vi "ConvertTEDtoWFM.vi"(9 "TED Status":T2[](array[typedef])=[{"Output"=FALSE, "SetPoint"=0.0, "Temperature"=0.0, "Current"=0.0, "Voltage"=0.0, "CableTrip"=FALSE, "TransducerTrip"=FALSE, "OverTemp"=FALSE}, {"Output"=FALSE, "SetPoint"=0.0, "Temperature"=0.0, "Current"=0.0, "Voltage"=0.0, "CableTrip"=FALSE, "TransducerTrip"=FALSE, "OverTemp"=FALSE}], 11 "Input cluster":T1) -> (1 "TED":waveform(dbl)[](graph), 3 "TED_Wfm":T1)   [LabVIEW 2025]
uses:
  controls/TED4015 Status.ctl
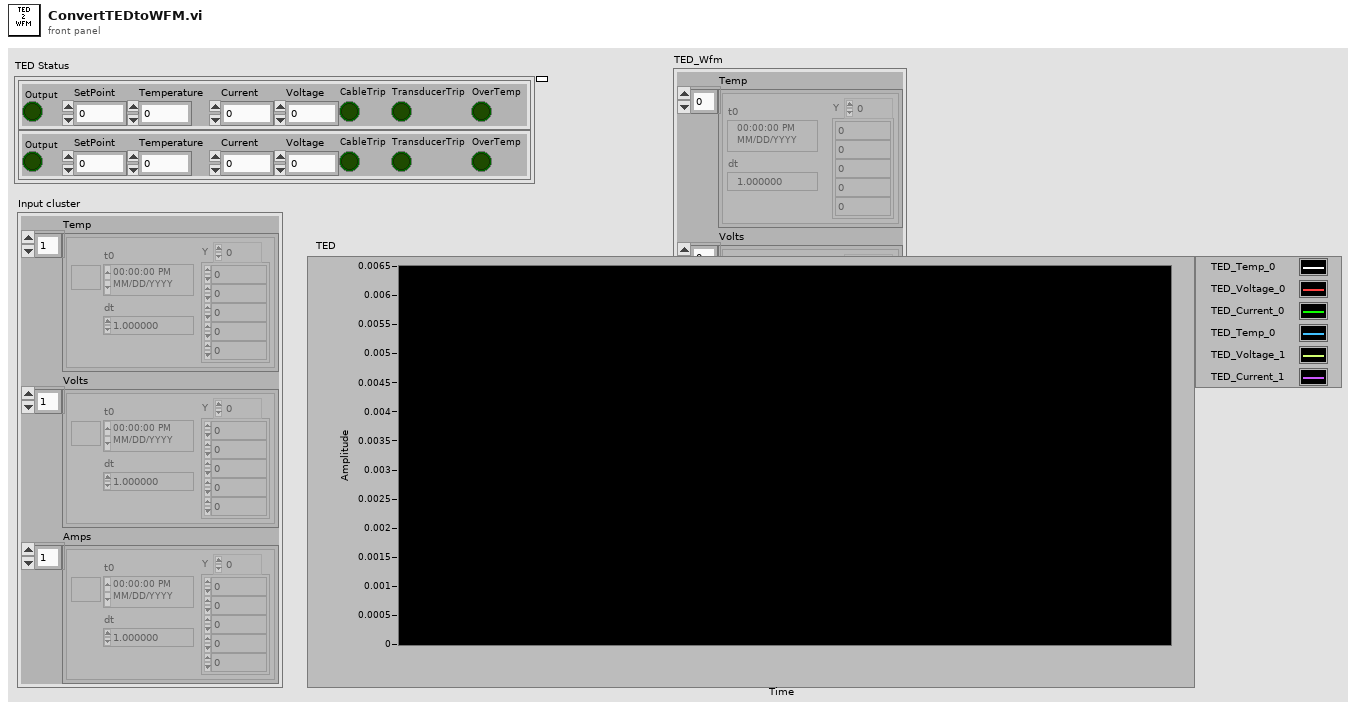
[diagram p1: front panel]
types:
  T1 = cluster{"Temp":waveform(dbl)[], "Volts":waveform(dbl)[], "Amps":waveform(dbl)[]}
  T2 = typedef "TED4015 Status.ctl" = cluster{"Output":bool, "SetPoint":dbl, "Temperature":dbl, "Current":dbl, "Voltage":dbl, "CableTrip":bool, "TransducerTrip":bool, "OverTemp":bool}
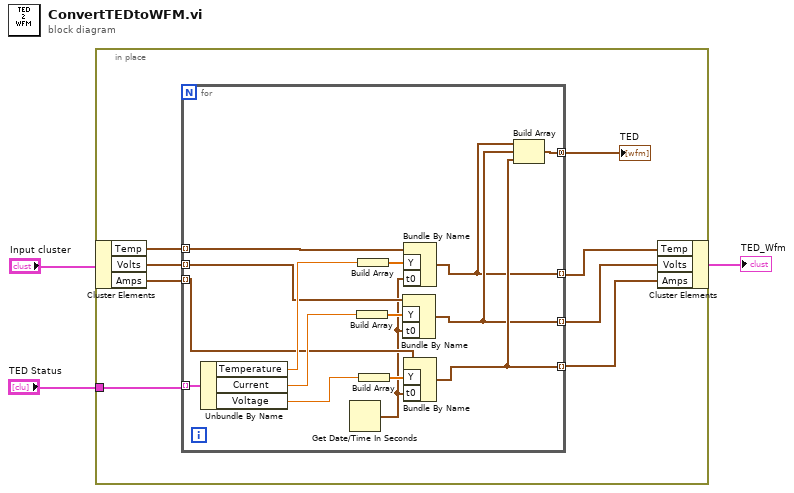
[diagram p0: block diagram]
diagram:
  n1 = in-place {
    in-place-border: "TED Status" -> [w5]
    n2 = in-place-cluster #1("Input cluster") -> ("Temp"=w11:waveform(dbl)[], "Volts"=w9:waveform(dbl)[], "Amps"=w7:waveform(dbl)[])
    n3 = for {
      tunnel: w5 -> [w26] mode=indexing
      tunnel: w11 -> [w17] mode=indexing
      tunnel: w9 -> [w18] mode=indexing
      tunnel: w7 -> [w19] mode=indexing
      tunnel: [w12] -> w10 mode=indexing
      tunnel: [w13] -> w8 mode=indexing
      tunnel: [w14] -> w6 mode=indexing
      tunnel: [w16] -> w4 mode=concatenating
      n4 = Unbundle By Name(w26) -> ("Temperature"=w25:dbl, "Current"=w21:dbl, "Voltage"=w20:dbl)
      n5 = Get Date/Time In Seconds() -> (seconds since 1Jan1904=w15:timestamp)
      n6 = Build Array(w21) -> (w23:dbl[])
      n7 = Build Array(w25) -> (w24:dbl[])
      n8 = Build Array(w20) -> (w22:dbl[])
      n9 = Bundle By Name(cluster=w18, "Y"=w23, "t0"=w15) -> (w13:waveform(dbl))
      n10 = Bundle By Name(cluster=w17, "Y"=w24, "t0"=w15) -> (w12:waveform(dbl))
      n11 = Bundle By Name(cluster=w19, "Y"=w22, "t0"=w15) -> (w14:waveform(dbl))
      n12 = Build Array(w12, w13, w14) -> (w16:waveform(dbl)[])
    }
    "TED" <- w4
    n13 = in-place-cluster #1("Temp"=w10, "Volts"=w8, "Amps"=w6) -> (→"TED_Wfm":T1)
  }
